vi "niLvFpga_Close_cRIO-9035 (Sync).vi"(0 "session in":u32, 5 "reset if last session (f)":bool, 11 "error in":errorcluster) -> (15 "error out":errorcluster)   [LabVIEW 2020]
uses:
  <vilib>/rvi/interface/common/niFpgaWaitOnOcc.vi
  NiFpgaLv.dll
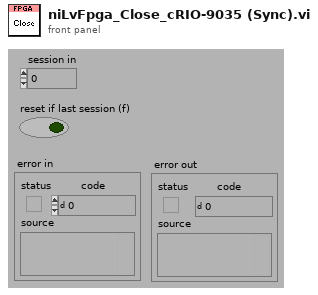
[diagram p1: front panel]
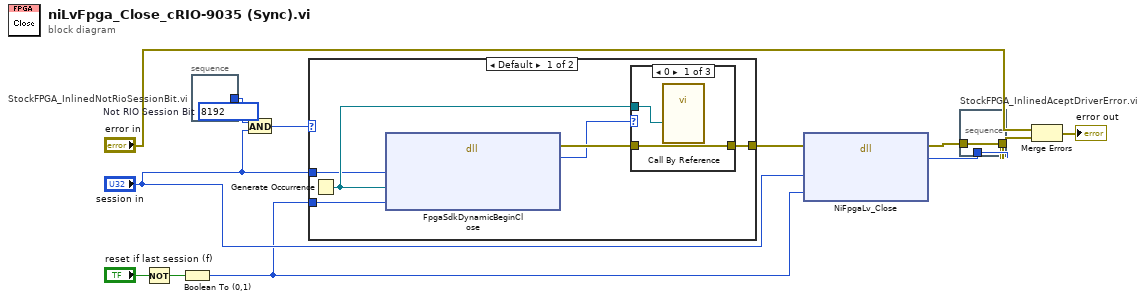
[diagram p0: block diagram]
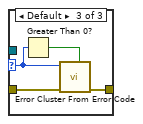
[diagram p4: hidden frame]
diagram:
  n1 = Not(x="reset if last session (f)") -> (.not. x?=w7:bool)
  n2 = Boolean To (0,1)(Boolean=w7) -> (0, 1=w3:i16)
  n3 = stacked-sequence "StockFPGA_InlinedNotRioSessionBit.vi" {
    tunnel: [w13] -> w6
    frame #0 {
      w13 = u32 8192  # Not RIO Session Bit
    }
  }
  n4 = And(x=w6, y="session in") -> (x .and. y?=w5:u32)
  n5 = case shown="Default" w5 {
    tunnel: [w16 _] -> w1
    tunnel: "session in" -> [w15 _]
    tunnel: w3 -> [w14 _]
    frame Default {
      n6 = Generate Occurrence() -> (w19:refnum<k4>)
      n7 = dll-call lib="LabVIEW" fn="FpgaSdkDynamicBeginClose"("session"=w15, "occurrence"=w19, "noResetIfLastSession"=w14) -> (error out=w18:errorcluster, "status"=w17:i32)  [unwired: 6 in, 1 out]
      n8 = case shown="0" w17 {
        selector: w17 -> [_ _ w23]
        tunnel: [w21 w22 w25] -> w16
        tunnel: w18 -> [w21 w22 w26]
        tunnel: w19 -> [w20 _ _]
        frame 0 {
          n9 = call-by-ref "?"("occurrence"=w20) -> ()  [unwired: 16 in, 3 out]
        }
        frame -61167 {
          # "emulation case intentionally ignoring error"
        }
        frame Default {
          n10 = Greater Than 0?(x=w23) -> (x > 0?=w24:bool)
          n11 = call <vilib>:"Error Cluster From Error Code.vi"("is warning? (False)"=w24, "error in (no error)"=w26, "error code (0)"=w23) -> ("error out"=w25:errorcluster)  [unwired: 6 in]
        }
      }
    }
    frame 0 {
    }
  }
  n12 = dll-call lib="NiFpgaLv.*" fn="NiFpgaLv_Close" label="niLvFpgaClose"(error in=w1, "sessionID"="session in", "noResetIfLastSession"=w3) -> (error out=w11:errorcluster, "status"=w10:i32)  [unwired: 3 in, 2 out]
  n13 = stacked-sequence "StockFPGA_InlinedAceptDriverError.vi" {
    tunnel: w11 -> [w27]
    tunnel: w10 -> [w29]
    tunnel: [w28] -> w8
    frame #0 {
      n14 = case shown="Default" w29 {
        selector: w29 -> [_ w31]
        tunnel: [w30 w33] -> w28
        tunnel: w27 -> [w30 w34]
        frame 0 {
        }
        frame Default {
          n15 = Greater Than 0?(x=w31) -> (x > 0?=w32:bool)
          n16 = call <vilib>:"Error Cluster From Error Code.vi"("is warning? (False)"=w32, "error in (no error)"=w34, "error code (0)"=w31) -> ("error out"=w33:errorcluster)  [unwired: 6 in]
        }
      }
    }
  }
  n17 = Merge Errors("error in", w8) -> (→"error out":errorcluster)
